vi "2D Normal Vector.vi"(4 "2D Vector":T1) -> (1 "2D Normal":T1)   [LabVIEW 2011]
uses:
  LIDAR Acquisition Loop/Simulation/2D Point.ctl
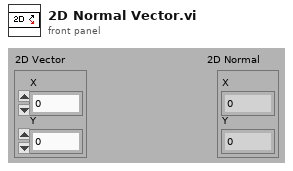
[diagram p1: front panel]
types:
  T1 = typedef "2D Point.ctl" = cluster{"X":dbl, "Y":dbl}
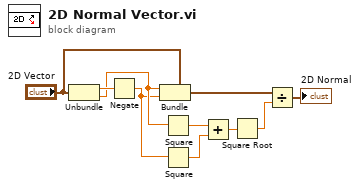
[diagram p0: block diagram]
diagram:
  n1 = Unbundle("2D Vector") -> ("X"=w9:dbl, "Y"=w8:dbl)
  n2 = Negate(x=w9) -> (-x=w7:dbl)
  n3 = Bundle(cluster="2D Vector", "X"=w8, "Y"=w7) -> (w2:T1)
  n4 = Square(x=w8) -> (x^2=w6:dbl)
  n5 = Square(x=w7) -> (x^2=w5:dbl)
  n6 = Add(x=w6, y=w5) -> (x+y=w4:dbl)
  n7 = Square Root(x=w4) -> (sqrt(x)=w3:dbl)
  n8 = Divide(x=w2, y=w3) -> (x/y=→"2D Normal":T1)
